vi "run.vi"(8 "error in (no error)":errorcluster, 11 "Controller in":refnum<class "Controller.lvclass">) -> (0 "error out":errorcluster, 3 "Controller out":refnum<class "Controller.lvclass">)   [LabVIEW 2016, in "Controller.lvclass"]
uses:
  Controller.lvclass
  Controller.lvclass/Controller.ctl
  UserEvents/UserEvents.lvclass/UserEvents.ctl
  Commands/Command/Command.lvclass
  UserEvents/UserEvents.lvclass
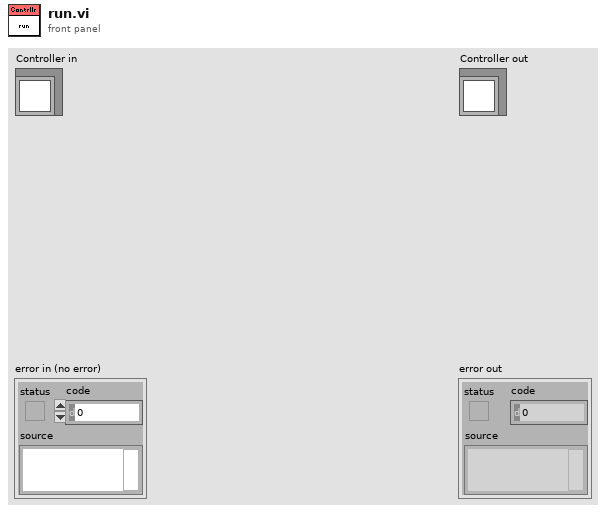
[diagram p1: front panel]
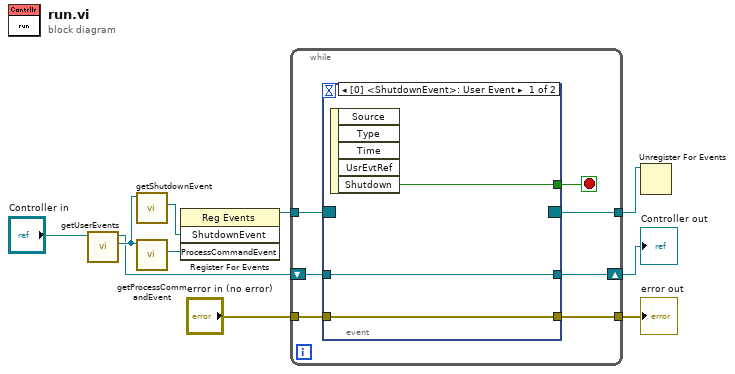
[diagram p0: block diagram]
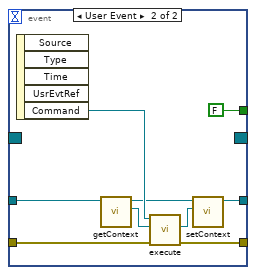
[diagram p2: hidden frame]
diagram:
  n1 = call "getUserEvents.vi"("Controller in"="Controller in") -> ("UserEvents"=w5:refnum<class "UserEvents.lvclass">, "Controller out"=w3:refnum<class "Controller.lvclass">)  [unwired: 9 in]
  n2 = call "getShutdownEvent.vi"("UserEvents in"=w5) -> ("ShutdownEvent"=w2:refnum<user-event>)  [unwired: 9 in, 1 out]
  n3 = call "getProcessCommandEvent.vi"("UserEvents in"=w5) -> ("ProcessCommandEvent"=w1:refnum<user-event>)  [unwired: 9 in, 1 out]
  n4 = register-events(w2, w1) -> (reference out=w10:refnum<event-registration>)  [unwired: 2 in, 1 out]
  n5 = while {
    tunnel: w10 -> [w17]
    shift-right: [w15] -> w9
    shift-left: w3 -> [w16]
    tunnel: [w14] -> w8
    tunnel: [w13] -> w6
    tunnel: "error in (no error)" -> [w12]
    stop <- w11 stop-if-true
    n6 = event shown="[0] <ShutdownEvent>: User Event" {
      selector: w17 -> [_ _]
      dyn-events: [_ _] -> w14
      timeout: _ -> [_ _]
      tunnel: w16 -> [w19 w29]
      tunnel: [w19 w24] -> w15
      tunnel: [w18 w23] -> w13
      tunnel: w12 -> [w18 w22]
      tunnel: [w20 FALSE ("Boolean")] -> w11
      event User Event {
        n7 = event-data() -> ("Shutdown"=w20:bool)  [unwired: 1 in, 4 out]
      }
      event User Event {
        n8 = event-data() -> ("Command"=w28:refnum<class "Command.lvclass">)  [unwired: 1 in, 4 out]
        n9 = call "getContext.vi"("Controller in"=w29) -> ("Context"=w27:refnum<class "Context.lvclass">, "Controller out"=w25:refnum<class "Controller.lvclass">)  [unwired: 9 in]
        n10 = call-dynamic "execute.vi"("error in (no error)"=w22, "Context in"=w27, "Command in"=w28) -> ("error out"=w23:errorcluster, "Context out"=w26:refnum<class "Context.lvclass">)  [unwired: 6 in, 1 out]
        n11 = call "setContext.vi"("Context"=w26, "Controller in"=w25) -> ("Controller out"=w24:refnum<class "Controller.lvclass">)  [unwired: 9 in]
      }
    }
  }
  "error out" <- w6
  "Controller out" <- w9
  n12 = Unregister For Events(event registration refnum=w8) -> ()  [unwired: 1 in, 1 out]
